vi "Measurement.OnEscaped.vi"(8 "error in (no error)":errorcluster, 10 "Escaped":T1, 11 "Measurement in":refnum<class "Measurement.lvclass">) -> (0 "error out":errorcluster, 3 "Measurement out":refnum<class "Measurement.lvclass">)   [LabVIEW 2017, in "Measurement.lvclass"]
uses:
  Measurement.lvclass
  Typedefs/PublicEvents--Measurement.Escaped.ctl
  Measurement.lvclass/Measurement.ctl
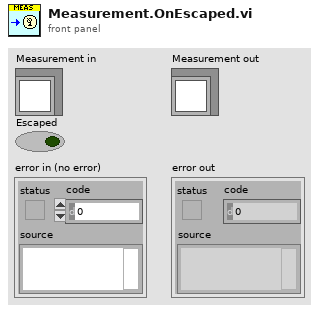
[diagram p1: front panel]
types:
  T1 = typedef "Measurement.lvclass/PublicEvents--Measurement.Escaped.ctl" = bool
  T2 = typedef "Measurement.lvclass/PrivateData--Ref.ctl" = refnum<data-value>
  T3 = typedef "Measurement.lvclass/PrivateData--Cluster.ctl" = cluster{"Public Events":T4, "Protected Events":T5}
  T4 = typedef "Measurement.lvclass/PublicEvents--Cluster.ctl" = cluster{"Initialized":refnum<user-event>, "Configured":refnum<user-event>, "Measured":refnum<user-event>, "Finished":refnum<user-event>, "Escaped":refnum<user-event>, "Uninitialized":refnum<user-event>}
  T5 = typedef "Measurement.lvclass/ProtectedEvents--Cluster.ctl" = cluster{"Initialize":refnum<user-event>, "Begin":refnum<user-event>, "Pause":refnum<user-event>, "End":refnum<user-event>, "Uninitialize":refnum<user-event>}
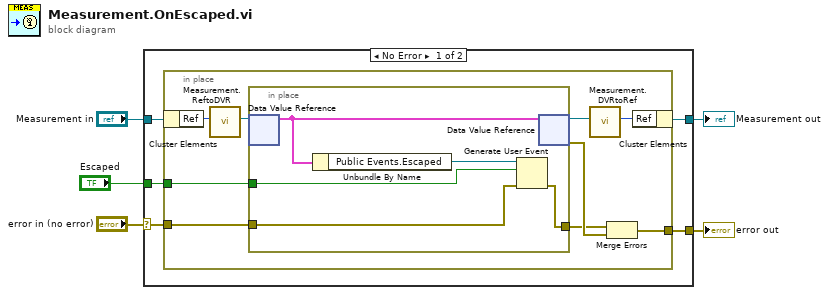
[diagram p0: block diagram]
diagram:
  n1 = case shown="No Error" "error in (no error)" {
    selector: "error in (no error)" -> [w9 w26]
    tunnel: [w8 w26] -> w4
    tunnel: [w7 w25] -> w2
    tunnel: "Measurement in" -> [w10 w25]
    tunnel: "Escaped" -> [w6 _]
    frame No Error {
      n2 = in-place {
        in-place-border: [w14] -> w8
        in-place-border: w9 -> [w13]
        in-place-border: w6 -> [w11]
        n3 = in-place-cluster #1(w10) -> ("Ref"=w19:u32)
        n4 = call "Measurement.ReftoDVR.vi"("Ref"=w19) -> ("Ref"=w18:T2)  [unwired: 10 in]
        n5 = in-place {
          in-place-border: w13 -> [w22]
          in-place-border: [w21] -> w12
          in-place-border: w11 -> [w20]
          n6 = in-place-dvr #2(w18) -> (w23:T3)  [unwired: 1 out]
          n7 = Unbundle By Name(w23) -> ("Public Events.Escaped"=w24:refnum<user-event>)
          n8 = Generate User Event(user event=w24, event data cluster=w20, error in=w22) -> (error out=w21:errorcluster)  [unwired: 1 in, 1 out]
          n9 = in-place-dvr #2(w23) -> (w17:T2, w15:errorcluster)
        }
        n10 = call "Measurement.DVRtoRef.vi"("Ref"=w17) -> ("Ref"=w16:u32)  [unwired: 10 in]
        n11 = Merge Errors(w12, w15) -> (w14:errorcluster)
        n12 = in-place-cluster #1("Ref"=w16) -> (w7:refnum<class "Measurement.lvclass">)
      }
    }
    frame Error {
    }
  }
  "error out" <- w4
  "Measurement out" <- w2
